vi "Hardware trigger simulator.vi"(3 "State":u8(ring) items=["LOW", "HIGH"]) -> ()   [LabVIEW 2017]
panel:
  out "Low":bool
  out "High":bool
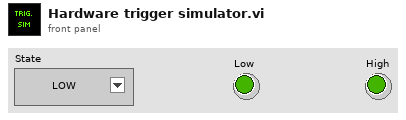
[diagram p1: front panel]
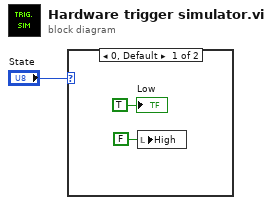
[diagram p0: block diagram]
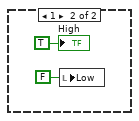
[diagram p2: hidden frame]
diagram:
  n1 = case shown="0, Default" "State" {
    frame 0, Default {
      n2 = local write "High"(FALSE ("High")) -> ()
      "Low" <- TRUE ("Low")
    }
    frame 1 {
      n3 = local write "Low"(FALSE ("Low")) -> ()
      "High" <- TRUE ("High")
    }
  }
